vi "Scale Waveform.vi"(6 "Variable Configuration":T1[](array[typedef]) {"Scaling"."Offset" format="%.5f"; "Scaling"."Gain" format="%.5f"; "Limits and responces"."Limits"."H" format="%.3f"; "Limits and responces"."Limits"."L" format="%.3f"; "Limits and responces"."Limits"."HH" format="%.3f"; "Limits and responces"."Limits"."LL" format="%.3f"}, 10 "Waveform":waveform(sgl), 11 "Var Tag":u16) -> (2 "output waveform":waveform(sgl))   [LabVIEW 2011]
doc: "This VI scales a waveform. The data buffer only provides unscaled data and hence this VI is necessary."
uses:
  User Setting Analog Channel Bg.ctl
  Scaling.ctl
  Alarm Setup Analog.ctl
  Alarm Responce.ctl
  Action List.ctl
  Limits.ctl
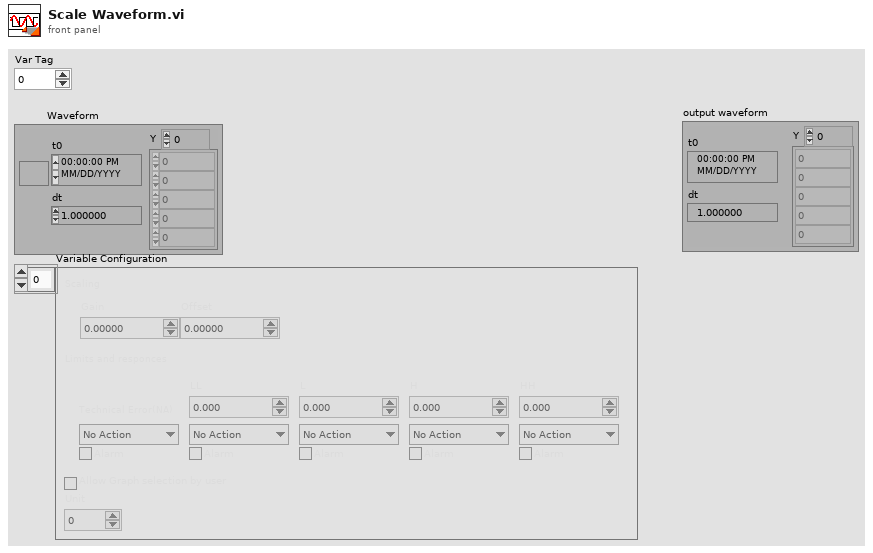
[diagram p1: front panel]
types:
  T1 = typedef "User Setting Analog Channel Bg.ctl" = cluster{"Scaling":T2, "Limits and responces":T3, "Allow Graph selection by user":bool, "Unit":u16}
  T2 = typedef "Scaling.ctl" = cluster{"Gain":dbl, "Offset":dbl}
  T3 = typedef "Alarm Setup Analog.ctl" = cluster{"Technical Error(NA)":T4, "LL":T4, "L":T4, "H":T4, "HH":T4, "Limits":T6}
  T4 = typedef "Alarm Responce.ctl" = cluster{"Action":T5, "Alarm":bool}
  T5 = typedef "Action List.ctl" = enum16{"No Action", "Stop Motor", "Turn Off HV"}
  T6 = typedef "Limits.ctl" = cluster{"LL":dbl, "L":dbl, "H":dbl, "HH":dbl}
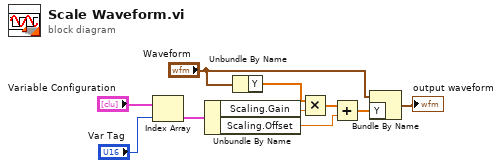
[diagram p0: block diagram]
diagram:
  n1 = Index Array(array="Variable Configuration", index="Var Tag") -> (element=w5:T1)
  n2 = Unbundle By Name(w5) -> ("Scaling.Gain"=w4:dbl, "Scaling.Offset"=w3:dbl)
  n3 = Unbundle By Name("Waveform") -> ("Y"=w8:sgl[])
  n4 = Multiply(x=w8, y=w4) -> (x*y=w7:dbl[])
  n5 = Add(x=w7, y=w3) -> (x+y=w6:dbl[])
  n6 = Bundle By Name(cluster="Waveform", "Y"=w6) -> (→"output waveform":waveform(sgl))
